vi "NML Analog Readout.vi"() -> ()   [LabVIEW 2024]
doc: "This VI is designed to scan the analog inputs and show the values on the screen. This can be used in repeat mode to be an 8 channel DVM.\nScott Hannahs, FBNML, April 1992"
uses:
  <vilib>/Utility/error.llb/DialogType.ctl
  <vilib>/_DAQmxBase/Internals/DAQmxBase Create Channel (AI-Voltage-Basic).vi
  <vilib>/_DAQmxBase/Internals/DAQmxBase Timing (Sample Clock).vi
  <vilib>/_DAQmxBase/Internals/DAQmxBase Read (Analog 2D DBL NChan NSamp).vi
  <vilib>/Analysis/NI_AALBase.lvlib
  <vilib>/Analysis/baseanly.llb/Mean (DBL).vi
panel:
  in  "stop":bool
  in  "Bipolar":bool
  in  "CHANNEL & RANGE SELECTOR":T1={"0"=3, "1"=4, "2"=0, "3"=0, "4"=0, "5"=0, "6"=0, "7"=0} {"0" scale=0.0..4.0; "7" scale=0.0..4.0; "6" scale=0.0..4.0; "5" scale=0.0..4.0; "4" scale=0.0..4.0; "3" scale=0.0..4.0; "2" scale=0.0..4.0; "1" scale=0.0..4.0}
  out "?":string="\r\r   \r \r\r"
  in  "Points Averaged":i32=32 min=3 max=32000
  # "Monopolar"
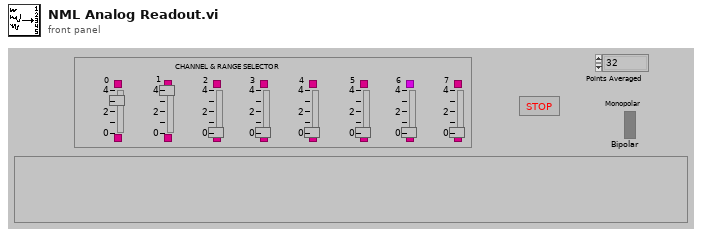
[diagram p1: front panel]
types:
  T1 = cluster{"0":i16, "1":i16, "2":i16, "3":i16, "4":i16, "5":i16, "6":i16, "7":i16}
  T2 = typedef "DialogType.ctl" = u16
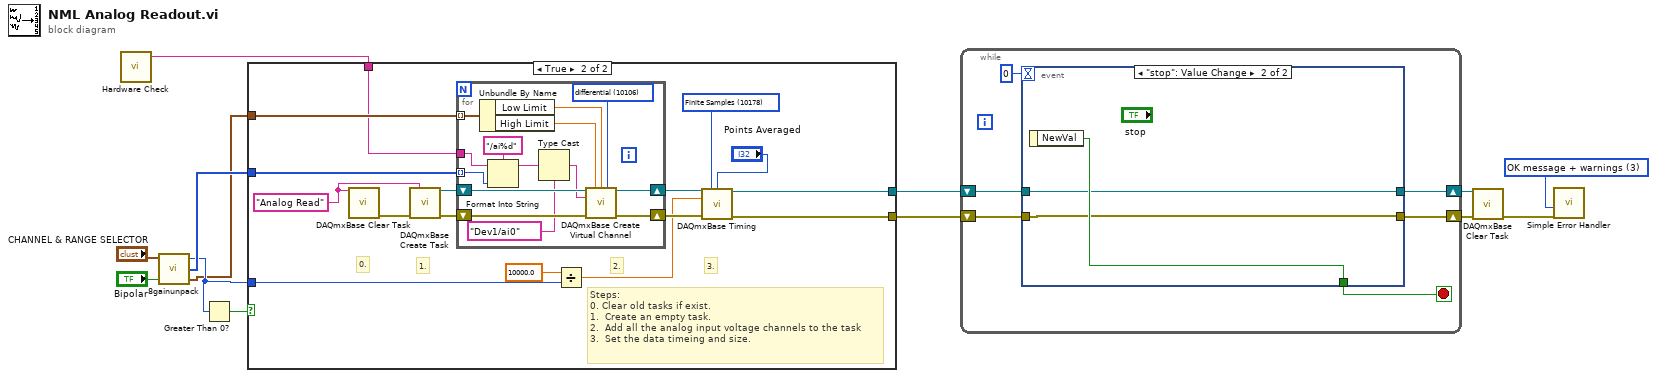
[diagram p0: block diagram]
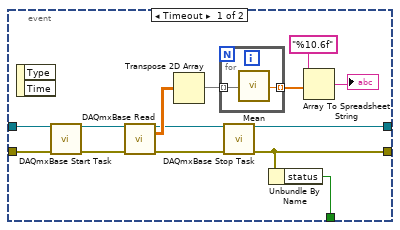
[diagram p2: hidden frame]
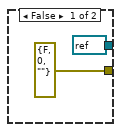
[diagram p3: hidden frame]
diagram:
  w3 = T2 3 items=["no dialog", "OK message", "continue or stop message", "OK message + warnings", "continue/stop + warnings"] ("type of dialog (OK msg:1)")
  n1 = call "Hardware Check.vi"() -> ("Data Acq Device"=w7:string)  [unwired: 1 in, 2 out]
  n2 = call "8gainunpack.vi"("GAIN & CHANNEL SELECTOR"="CHANNEL & RANGE SELECTOR", "Monopolar"="Bipolar") -> ("Number of channels"=w9:i32, "channels (0)"=w11:i32[], "Input Limits"=w8:cluster{"High Limit":dbl, "Low Limit":dbl}[])
  n3 = Greater Than 0?(x=w9) -> (x > 0?=w10:bool)
  n4 = case shown="True" w10 {
    tunnel: [errorcluster {"status"=FALSE, "code"=0, "source"=""} ("error out") w26] -> w5
    tunnel: [refnum<k21> refnum ("task out") w25] -> w6
    tunnel: w11 -> [_ w24]
    tunnel: w9 -> [_ w20]
    tunnel: w8 -> [_ w19]
    tunnel: w7 -> [_ w18]
    frame False {
    }
    frame True {
      w23 = "Analog Read" ("new task name")
      w27 = 10178 items=["Finite Samples"=10178, "Continuous Samples"=10123, "Hardware Timed Single Point"=12522] ("sample mode")
      # "0."
      # "3."
      # "2."
      # "1."
      # "Steps: \n0. Clear old tasks if exist.\n1.  Create an empty task.\n2.  Add all the analog input voltage channels to the task\n3.  Set the data timeing and size."
      n5 = call <vilib>:"DAQmxBase Clear Task.vi"("task in"=w23) -> ("error out"=w22:errorcluster)  [unwired: 14 in]
      n6 = call <vilib>:"DAQmxBase Create Task.vi"("new task name"=w23, "error in"=w22) -> ("task out"=w31:refnum<k21>, "error out"=w30:errorcluster)  [unwired: 12 in]
      n7 = for {
        tunnel: w19 -> [w45] mode=indexing
        tunnel: w24 -> [w37] mode=indexing
        shift-right: [w42] -> w29
        shift-left: w31 -> [w44]
        shift-right: [w41] -> w28
        shift-left: w30 -> [w43]
        tunnel: w18 -> [w36]
        w32 = 10106 items=["default"=-1, "differential"=10106, "RSE"=10083, "NRSE"=10078] ("input terminal configuration")
        n8 = Unbundle By Name(w45) -> ("Low Limit"=w40:dbl, "High Limit"=w39:dbl)
        n9 = Format Into String(format string="/ai%d", initial string=w36, w37) -> (resulting string=w38:string)  [unwired: 1 in, 1 out]
        n10 = Type Cast(type=tag "Dev1/ai0" ("Physical Channel 2"), x=w38) -> (*(type *) &x=w34:tag)
        n11 = call-poly <vilib>:"DAQmxBase Create Virtual Channel.vi"("task in"=w44, "maximum value"=w39, "minimum value"=w40, "input terminal configuration"=w32, "physical channels"=w34, "error in"=w43) -> ("task out"=w42:refnum<k21>, "error out"=w41:errorcluster)  [unwired: 8 in]
      }
      n12 = Divide(x=10000.0, y=w20) -> (x/y=w21:dbl)
      n13 = call-poly <vilib>:"DAQmxBase Timing.vi"("task/channels in"=w29, "sample mode"=w27, "samples per channel"="Points Averaged", "rate"=w21, "error in"=w28) -> ("task out"=w25:refnum<k21>, "error out"=w26:errorcluster)  [unwired: 9 in]
    }
  }
  n14 = while {
    shift-right: [w48] -> w2
    shift-left: w6 -> [w50]
    shift-right: [w47] -> w1
    shift-left: w5 -> [w49]
    stop <- w46 stop-if-true
    n15 = event shown="[1] \"stop\": Value Change" {
      selector: _ -> [_ _]
      dyn-events: _ -> [_ _]
      timeout: 0 -> [_ _]
      tunnel: w50 -> [w56 w68]
      tunnel: w49 -> [w55 w69]
      tunnel: [w54 w68] -> w48
      tunnel: [w53 w69] -> w47
      tunnel: [w52 w70] -> w46
      event Timeout {
        n16 = event-data() -> ()  [unwired: 1 in, 2 out]
        n17 = call <vilib>:"DAQmxBase Start Task.vi"("task/channels in"=w56, "error in"=w55) -> ("task out"=w63:refnum<k21>, "error out"=w64:errorcluster)  [unwired: 12 in]
        n18 = call-poly <vilib>:"DAQmxBase Read.vi"("task/channels in"=w63, "error in"=w64) -> ("task out"=w61:refnum<k21>, "data"=w65:dbl[][], "error out"=w62:errorcluster)  [unwired: 11 in]
        n19 = Transpose 2D Array(2D array=w65) -> (transposed array=w60:dbl[][])
        n20 = for {
          tunnel: w60 -> [w67] mode=indexing
          tunnel: [w66] -> w59 mode=indexing
          n21 = call-poly <vilib>:"Mean.vi"("X"=w67) -> ("mean"=w66:dbl)  [unwired: 1 out]
        }
        n22 = call <vilib>:"DAQmxBase Stop Task.vi"("task/channels in"=w61, "error in"=w62) -> ("task out"=w54:refnum<k21>, "error out"=w53:errorcluster)  [unwired: 12 in]
        n23 = Unbundle By Name(w53) -> ("status"=w52:bool)
        n24 = Array To Spreadsheet String(array=w59, 3:"%10.6f") -> (spreadsheet string=→"?":string)  [unwired: 1 in]
      }
      event "stop": Value Change {
        n25 = event-data() -> ("NewVal"=w70:bool)  [unwired: 1 in]
      }
    }
  }
  n26 = call <vilib>:"DAQmxBase Clear Task.vi"("task in"=w2, "error in"=w1) -> ("error out"=w4:errorcluster)  [unwired: 13 in]
  n27 = call <vilib>:"Simple Error Handler.vi"("type of dialog (OK msg:1)"=w3, "error in (no error)"=w4) -> ()  [unwired: 3 in, 5 out]
